vi "Tubing_Corrections_17.vi"() -> (5 "Plug in titles":string[](array[string]), 7 "Plug in values":string[](array[string]))   [LabVIEW 2010]
uses:
  Globals/Meas_global.vi
  <vilib>/Analysis/NI_AALPro.lvlib
  <vilib>/Utility/file.llb/Read From Spreadsheet File (DBL).vi
  <vilib>/Analysis/2dsp.llb/Inverse Real FFT.vi
panel:
  in  "Use a Smoothed\nAverage ITF?":u16(ring) caption="Save Data?" items=["Yes", "No"]
  out "Analogue Out":dbl[][](array[numeric])
  in  "Analogue In":dbl[][](array[numeric])
  in  "Top Level Folder":path
  in  "Use a DC Mag. of 1?":u16(ring)=1 caption="Save Data?" items=["Yes", "No"]
  out "Maximum frequency used from ITF <= Frequency covered in ITF":bool
  in  "Max.  Freq. covered in ITF":dbl=10000.0
  out "No. of samples used is an even no.":bool
  in  "Transducer\nZero Reading":dbl format="%#_p"
  in  "Inv Trans Function":u16(ring) caption="Save Data?" items=["Lee", "RWDI"]
  out "Pressure Signal":cluster{"Y":dbl[], "Y":dbl[]}[](graph)
  out "No. of samples used is constant throughout":bool
  out "Frequency of data used = as taken from the ITF":bool
  out "No. of samples per block\ntaken from raw data":dbl
  in  "Max.  Freq. required from ITF":dbl=10000.0
  in  "Distorted Pressure Channel:":dbl=2.0
  out "No. of samples recorded in raw data = as requested":bool
  in  "Tube Length":u16(ring)=1800 items=["0 mm"=0, "1100 mm"=1100, "1200 mm"=1200, "1300 mm"=1300, "1400 mm"=1400, "1500 mm"=1500, "1600 mm"=1600, "1700 mm"=1700, "1800 mm"=1800, "1900 mm"=1900, "2000 mm"=2000, "2100 mm"=2100, "2200 mm"=2200, "2300 mm"=2300, "2400 mm"=2400, "2500 mm"=2500, "2600 mm"=2600, "2700 mm"=2700, "2800 mm"=2800]
  out "Processing last block?":bool
  # "PLUG IN VI TO APPLY THE INVERSE TRANSFER FUNCTION TO THE PRESSURE DATA COLLECTED."
  # "NOTE: The run/test that is used in the ITF is read from a spreadsheet file.  Therefore when the best ones are found they can be kept and easily accessed.  If the boxes here are left as zero then they will be ignored even if changing the ITF used."
  # "USER INPUTS:"
  # "NOTE: If an average ITF is being used then input the final block number included in the average in this space here.  If a smoothed average is being used then pit \"YES\" in both the average and smoothed inputs."
  # "NOTE: The first thing in the list in the measurement program is channel 0 and second is 1 etc..., regardless of the channel number on the ADC."
  # "NOTE: The frequency of the raw data collected needs to be a product of the maximum frequency used from the ITF file when a lower ITF frequency is used (probably 1000 Hz like in RWDI's) than that of the sampling frequency of the collected pressure.  This is so this 'plug-in' can easily take the number of samples required.  If all of the samples are required then input the sampling frequency as the frequency required from the ITF!"
  # "NOTE: The raw data to be corrected needs to be sent through an analogue low pass filter before being sent to the ADC.  This must be equal to or lower than the Nyquist frequency (half of the sampling frequency).  This will then determine the max. frequency that can be presented in the form of the spectrum."
  # "NUMBER OF VALUES USED IN SMOOTHING THE AVERAGE SPECTRA (FiOR THIS GRAPH ONLY!!)"
  # "NOTE: If you don't put all of the blocks in the same file then it won't try to append to old files"
  # "NOTE: If the transfer function is to be changed and the effect on the RMS and spectra is to be analysed then the user can append as many runs as they like to the RMS and Spectra files by altering the relevant input here."
  # "SAVE BLOCKS BETWEEN:"
  # "AND"
  # "OUTPUTS:"
  # "NOTE: If you only want one block, just put the block number in both of the boxes shown here"
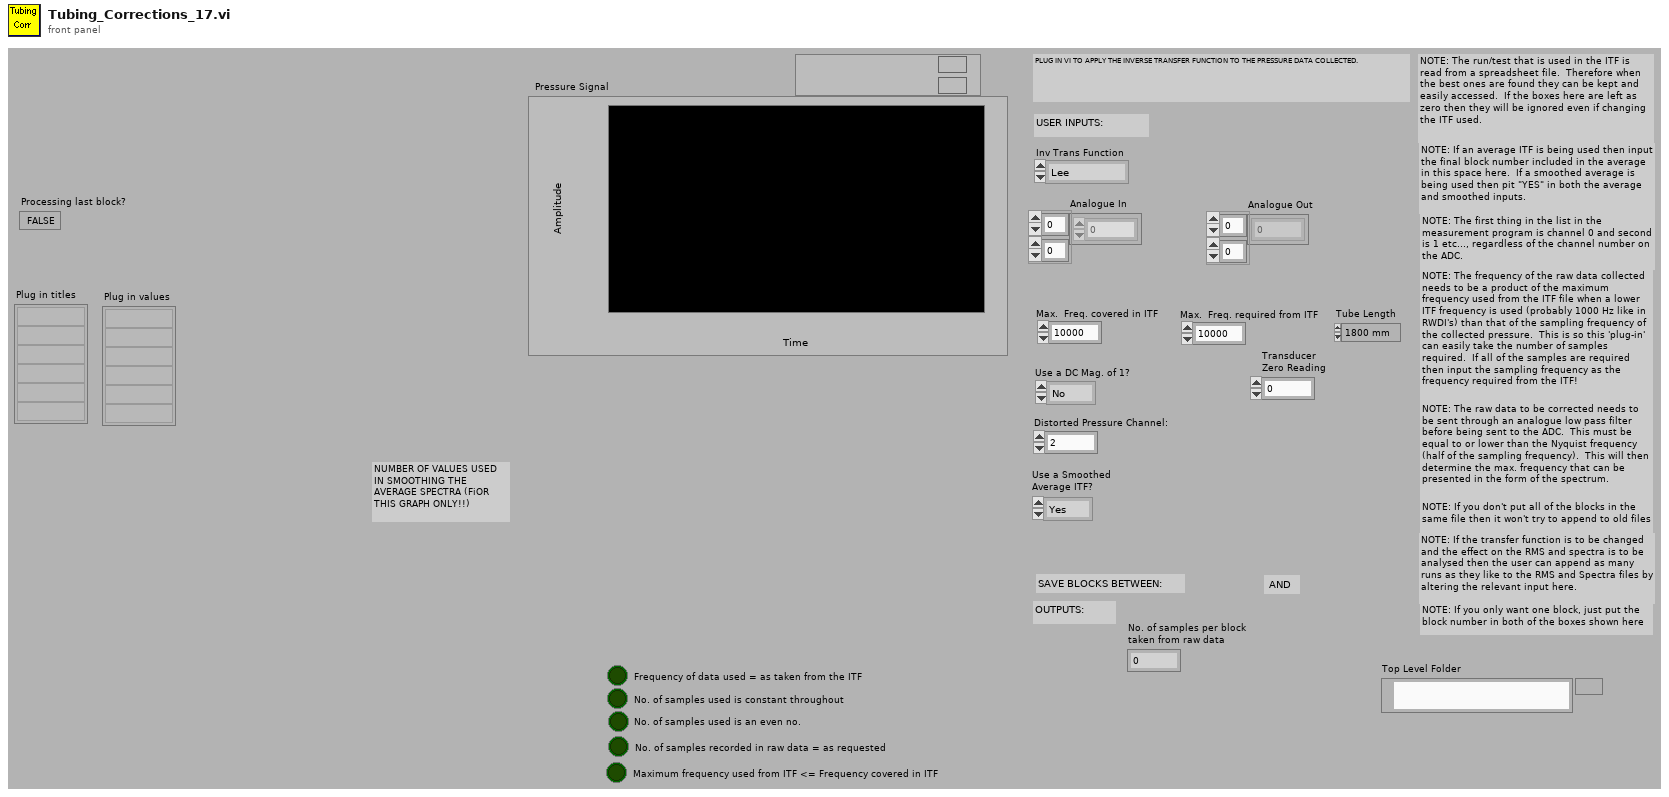
[diagram p1: front panel]
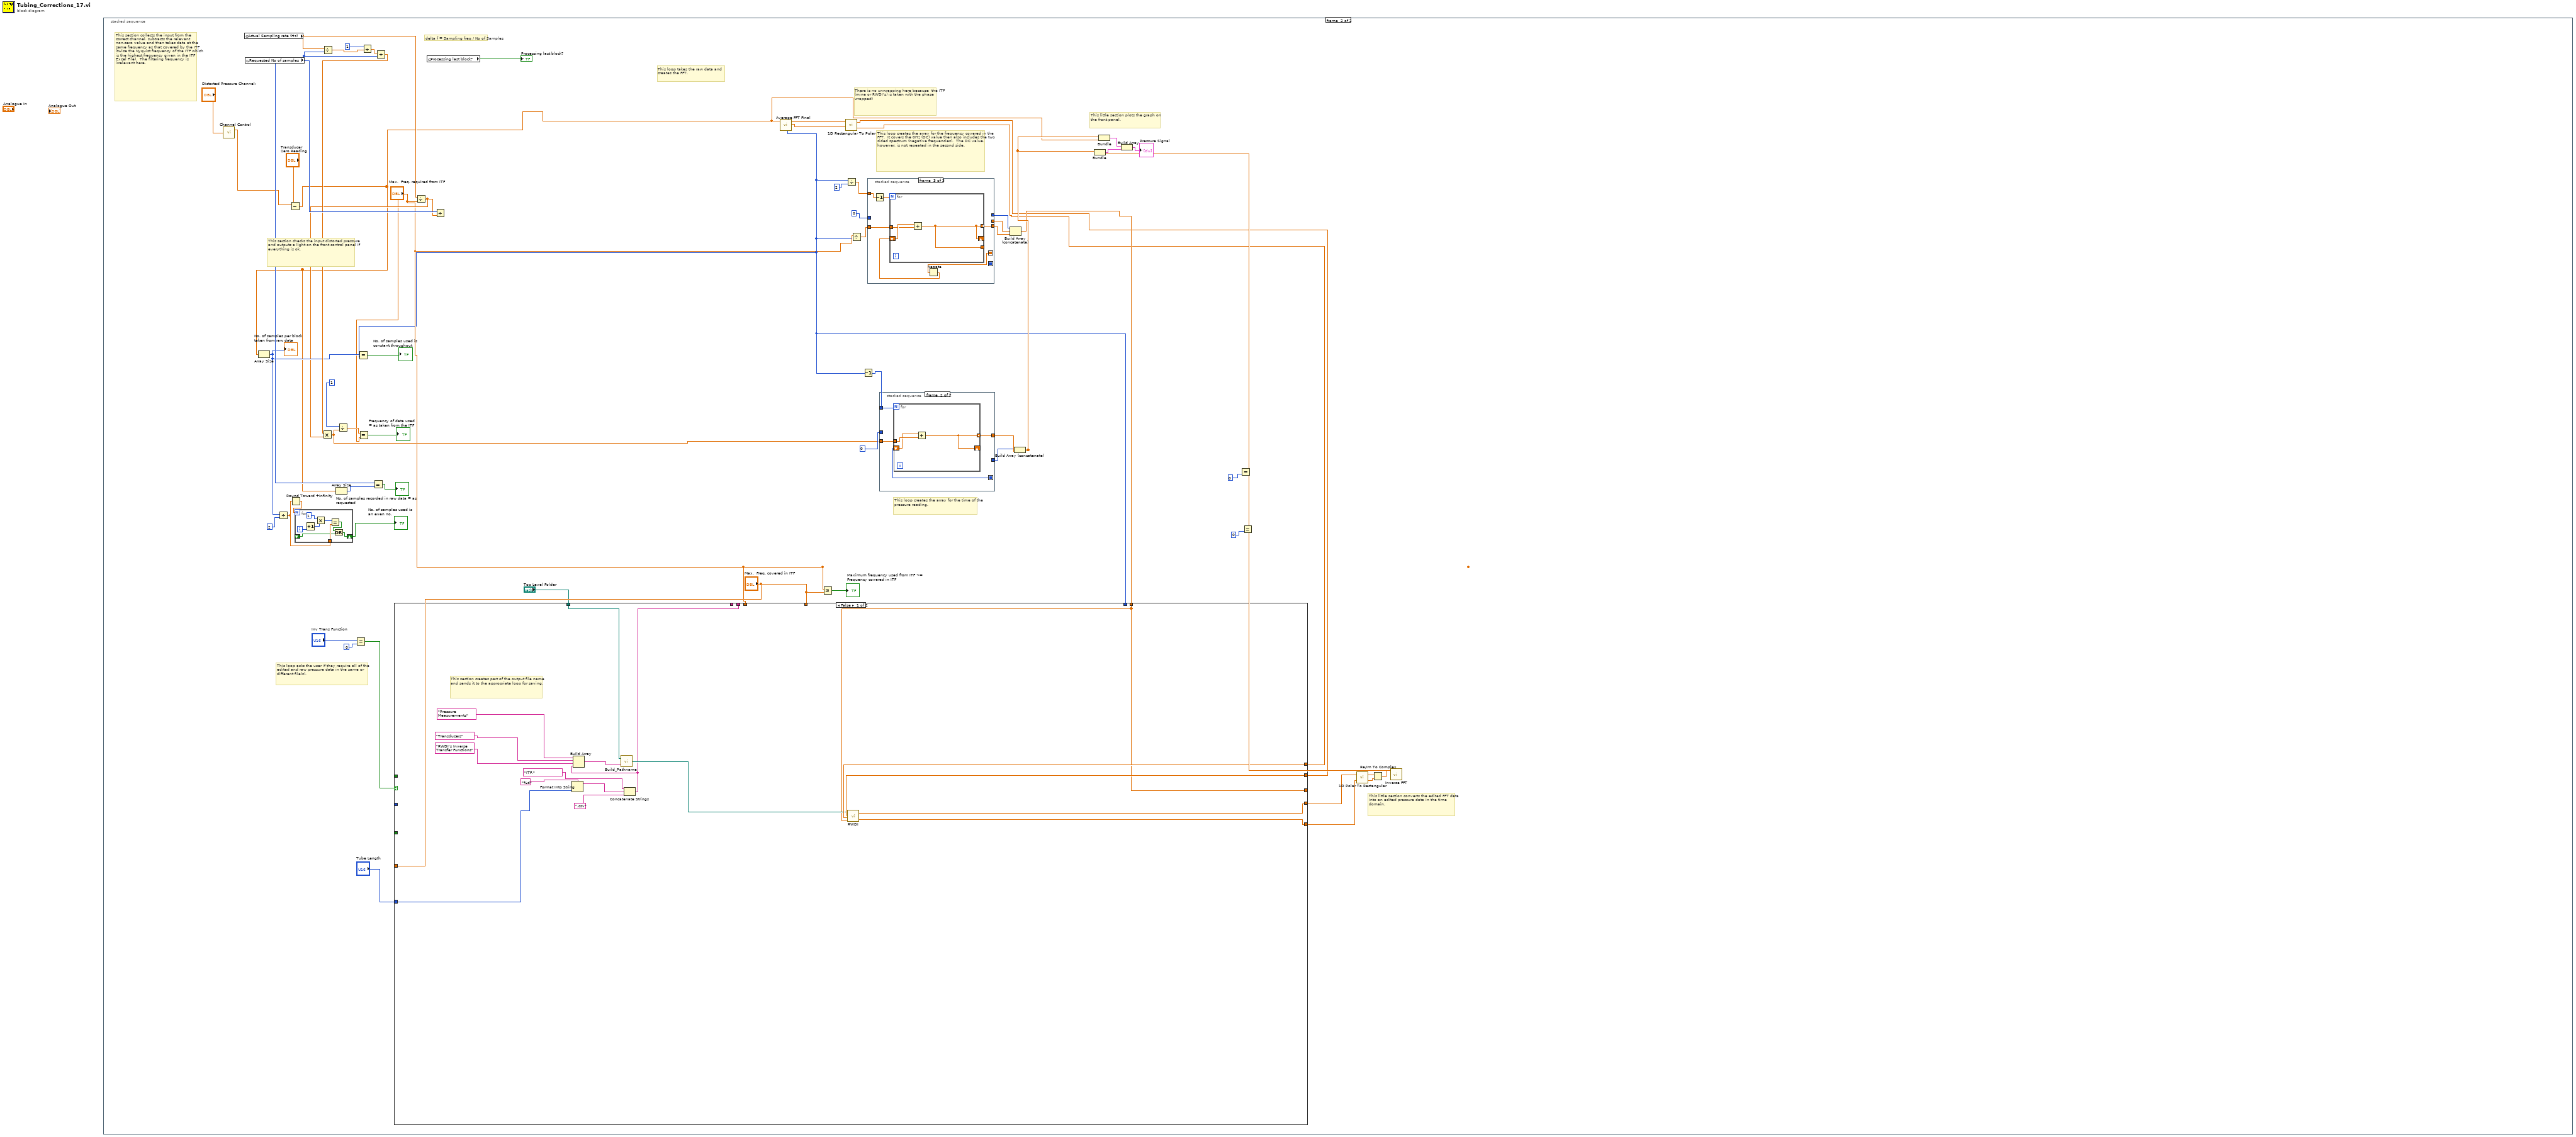
[diagram p0: block diagram]
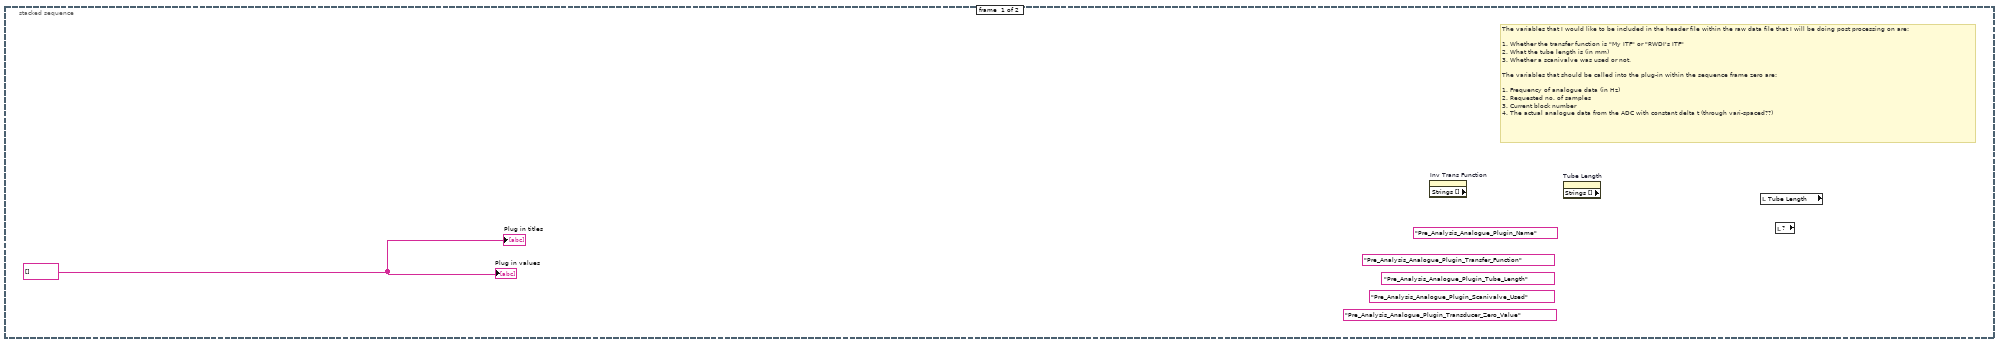
[diagram p2: hidden frame]
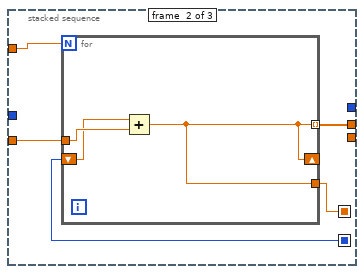
[diagram p4: hidden frame]
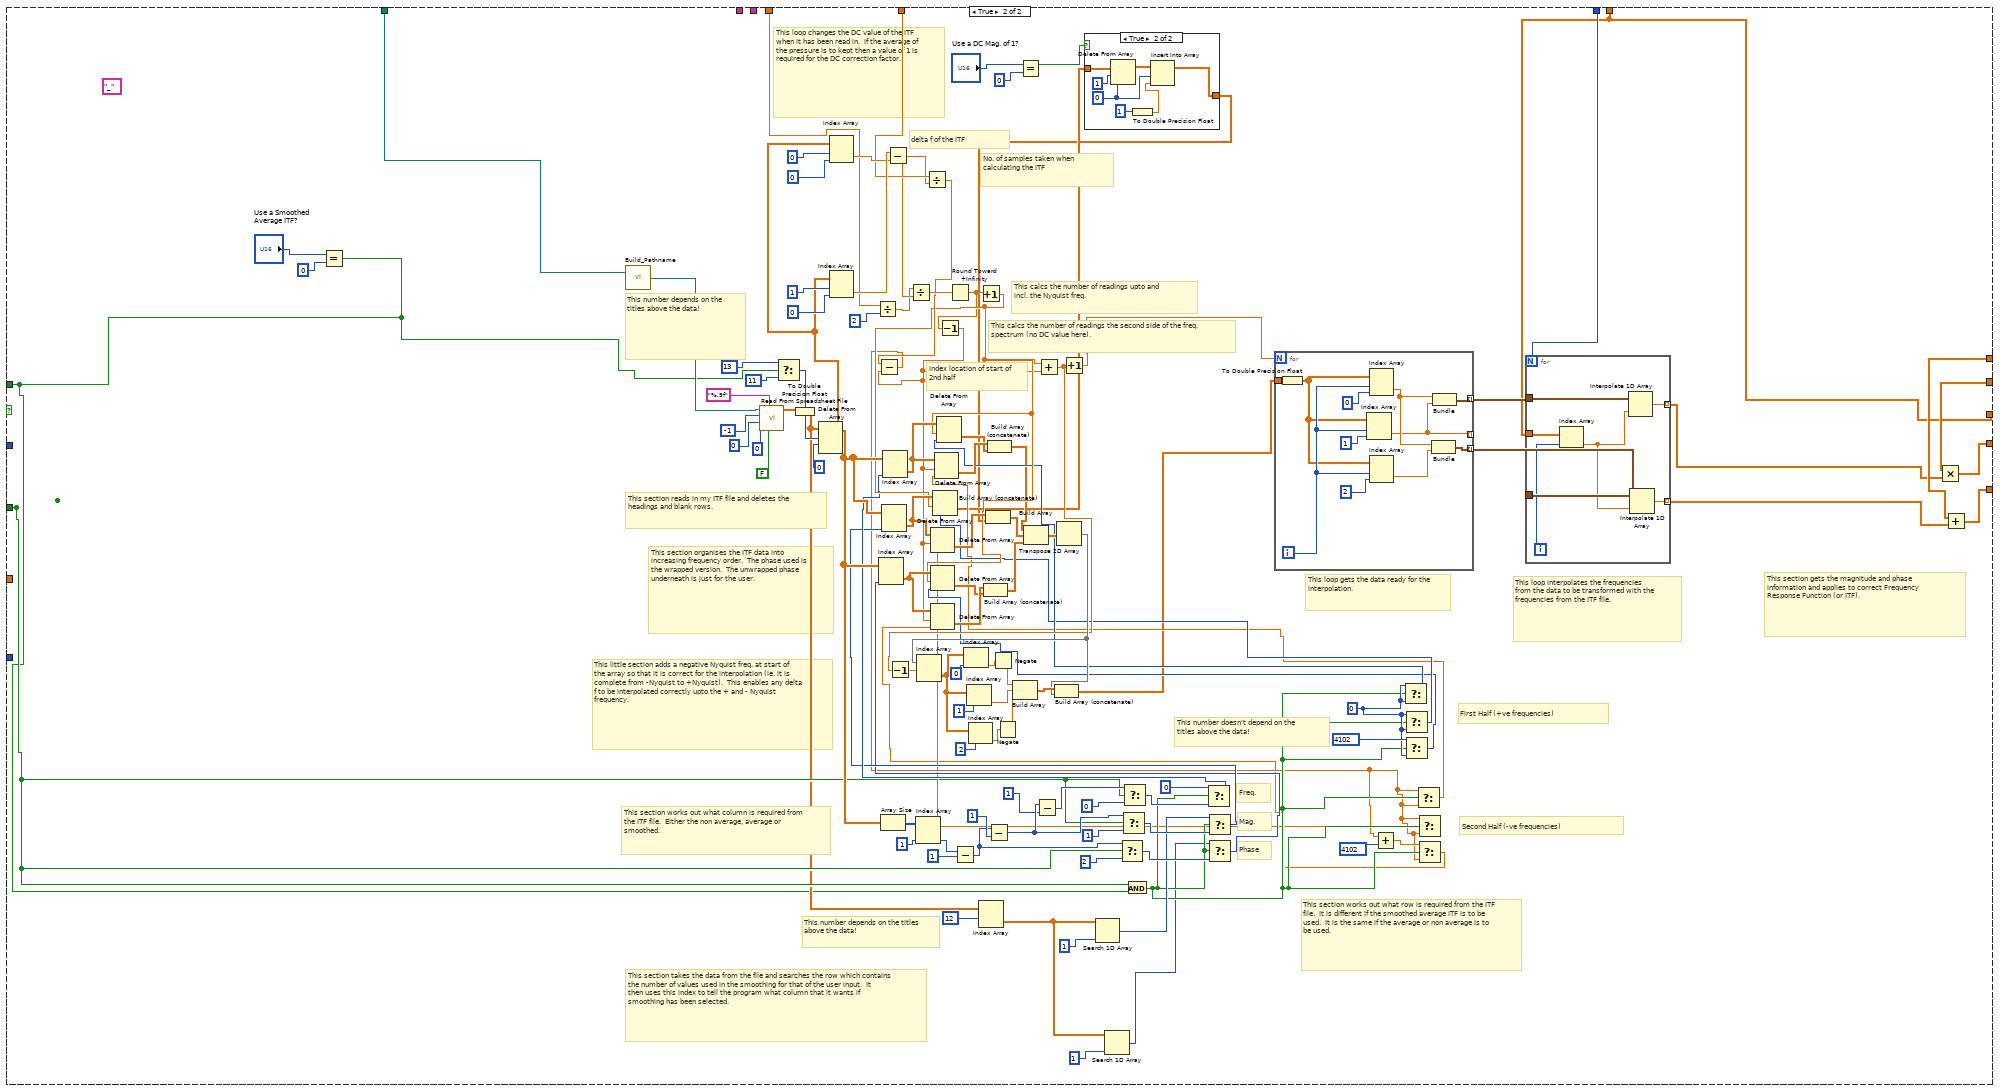
[diagram p5: hidden frame]
diagram:
  n1 = stacked-sequence {
    frame #0 {
      (unwired) "Pre_Analysis_Analogue_Plugin_Transducer_Zero_Value"
      (unwired) "Pre_Analysis_Analogue_Plugin_Scanivalve_Used"
      (unwired) "Pre_Analysis_Analogue_Plugin_Tube_Length"
      (unwired) "Pre_Analysis_Analogue_Plugin_Name"
      (unwired) "Pre_Analysis_Analogue_Plugin_Transfer_Function"
      w1 = string[] [] ("Add in values")
      # "The variables that I would like to be included in the header file within the raw data file that I will be doing post processing on are:\n\n1. Whether the transfer function is \"My ITF\" or \"RWDI's ITF\"\n2. What the tube length is (in mm)\n3. Whether a scanivalve was used or not.\n\nThe variables that should be called into the plug-in within the sequence frame zero are:\n\n1. Frequency of analogue data (in Hz)\n2. Requested no. of samples\n3. Current block number\n4. The actual analogue data from the ADC with constant delta t (through vari-spaced??)"
      n2 = property on="Inv Trans Function" class="Ring (strict)" props=["Strings []"]() -> ()  [unwired: 2 in, 3 out]
      n3 = property on="Tube Length" class="Ring (strict)" props=["Strings []"]() -> ()  [unwired: 2 in, 3 out]
      n4 = local read "Tube Length"() -> ()  [unwired: 1 out]
      n5 = local read item#-1() -> ()  [unwired: 1 out]
      "Plug in titles" <- w1
      "Plug in values" <- w1
    }
    frame #1 {
      # "This little section converts the edited FFT data into an edited pressure data in the time domain."
      # "There is no unwrapping here because  the ITF (mine or RWDI's) is taken with the phase wrapped!"
      # "This loop creates the array for the time of the pressure reading."
      # "This loop creates the array for the frequency covered in the FFT.  It covers the 0Hz (DC) value then also includes the two sided spectrum (negative frequencies).  The DC value, however, is not repeated in the second side."
      # "This loop takes the raw data and creates the FFT."
      # "This section collects the input from the correct channel, subtracts the relevant non-zero value and then takes data at the same frequency as that covered by the ITF (twice the Nyquist frequency of the ITF which is the highest frequency given in the ITF Excel File).  The filtering frequency is irrelevant here."
      # "This section checks the input distorted pressure and outputs a light on the front control panel if everything is ok."
      # "This little section plots the graph on the front panel."
      # "This loop asks the user if they require all of the edited and raw pressure data in the same or different file(s)."
      # "delta f = Sampling freq / No of Samples"
      n6 = call "Channel Control.vi"("Distorted Pressure Channel"="Distorted Pressure Channel:") -> ("Distorted Raw Data"=w10:dbl[])  [unwired: 1 out]
      n7 = global read "Meas_global.vi" "Actual Sampling rate (Hz)"() -> (w60:dbl)
      n8 = global read "Meas_global.vi" "Requested No of samples"() -> (w55:i32)
      n9 = Subtract(x=w10, y="Transducer\nZero Reading") -> (x-y=w5:dbl[])
      n10 = Array Size(array=w5) -> (size(s)=w23:i32)
      "No. of samples per block\ntaken from raw data" <- w23
      n11 = Divide(x=w23, y=2) -> (x/y=w24:dbl)
      n12 = Round Toward +Infinity(x=w24) -> (ceil(x): smallest int >= x=w27:dbl)
      n13 = for {
        N: w27 -> [_]
        tunnel: w24 -> [w75]
        shift-right: [w72] -> w26
        shift-left: _ -> [w73]
        i -> [w79]
        n14 = Increment(x=w79) -> (x+1=w78:i32)
        n15 = Multiply(x=1, y=w78) -> (x*y=w76:i32)
        n16 = Equal?(x=w76, y=w75) -> (x = y?=w74:bool)
        n17 = Or(x=w74, y=w73) -> (x .or. y?=w72:bool)
      }
      "No. of samples used is an even no." <- w26
      n18 = Divide(x=w60, y=w55) -> (x/y=w61:dbl)
      n19 = Array Size(array=w5) -> (size(s)=w54:i32)
      n20 = Equal?(x="Inv Trans Function", y=0) -> (x = y?=w36:bool)
      n21 = Divide(x=1, y=w61) -> (x/y=w59:dbl)
      n22 = Equal?(x=w55, y=w54) -> (x = y?=→"No. of samples recorded in raw data = as requested":bool)
      n23 = Divide(x=w59, y=w55) -> (x/y=w49:dbl)
      n24 = Divide(x=w60, y="Max.  Freq. required from ITF") -> (x/y=w21:dbl)
      n25 = Multiply(x=w49, y=w21) -> (x*y=w35:dbl)
      n26 = Divide(x=1, y=w35) -> (x/y=w57:dbl)
      n27 = Equal?(x=w57, y="Max.  Freq. required from ITF") -> (x = y?=→"Frequency of data used = as taken from the ITF":bool)
      n28 = global read "Meas_global.vi" "Processing last block?"() -> (→"Processing last block?":bool)
      n29 = Divide(x=w55, y=w21) -> ()  [unwired: 1 out]
      n30 = call "Average FFT Final.vi"("Distorted Pressure"=w5) -> ("Spectrum output Imaginary array"=w7:dbl[], "Spectrum output Real array"=w8:dbl[], "No of samples"=w6:i32)  [unwired: 7 in]
      n31 = Equal?(x=w23, y=w6) -> (x = y?=→"No. of samples used is constant throughout":bool)
      n32 = Less Or Equal?(x="Max.  Freq. required from ITF", y="Max.  Freq. covered in ITF") -> (x <= y?=→"Maximum frequency used from ITF <= Frequency covered in ITF":bool)
      n33 = call <vilib>:"1D Rectangular To Polar.vi"("X"=w8, "Y"=w7) -> ("Magnitude"=w3:dbl[], "Phase"=w2:dbl[])  [unwired: 1 out]
      n34 = Divide(x=w6, y=2) -> (x/y=w31:dbl)
      n35 = Divide(x="Max.  Freq. required from ITF", y=w6) -> (x/y=w33:dbl)
      n36 = Decrement(x=w6) -> (x-1=w66:i32)
      n37 = stacked-sequence {
        seq-local: [w80 _ _] -> [_ w84 _]
        seq-local: [_ w83 _] -> [_ _ w92]
        tunnel: 0 -> [w80 _ _]
        tunnel: w33 -> [_ w85 w94]
        tunnel: w31 -> [_ w82 w90]
        tunnel: [_ w81 _] -> w29
        tunnel: [w80 _ _] -> w30
        tunnel: [_ _ w93] -> w28
        frame #0 {
        }
        frame #1 {
          n38 = for {
            N: w82 -> [_]
            tunnel: w85 -> [w88]
            tunnel: [w86] -> w81 mode=indexing
            shift-right: [w86] -> _
            shift-left: w84 -> [w87]
            tunnel: [w86] -> w83
            n39 = Add(x=w87, y=w88) -> (x+y=w86:dbl)
          }
        }
        frame #2 {
          n40 = Decrement(x=w90) -> (x-1=w89:dbl)
          n41 = Negate(x=w92) -> (-x=w91:dbl)
          n42 = for {
            N: w89 -> [_]
            tunnel: [w95] -> w93 mode=indexing
            shift-right: [w95] -> _
            shift-left: w91 -> [w97]
            tunnel: [w95] -> _
            tunnel: w94 -> [w96]
            n43 = Add(x=w97, y=w96) -> (x+y=w95:dbl)
          }
        }
      }
      n44 = stacked-sequence {
        seq-local: [w257 _] -> [_ w258]
        tunnel: 0 -> [w257 _]
        tunnel: w35 -> [_ w260]
        tunnel: w66 -> [_ w261]
        tunnel: [_ w259] -> w65
        tunnel: [w257 _] -> w64
        frame #0 {
        }
        frame #1 {
          n45 = for {
            N: w261 -> [_]
            tunnel: w260 -> [w264]
            tunnel: [w263] -> w259 mode=indexing
            shift-right: [w263] -> _
            shift-left: w258 -> [w262]
            n46 = Add(x=w262, y=w264) -> (x+y=w263:dbl)
          }
        }
      }
      n47 = Build Array (concatenate)(w30, w29, w28) -> (w4:dbl[])
      n48 = case shown="False" w36 {
        tunnel: [_ w127] -> w22
        tunnel: w4 -> [w98 w120]
        tunnel: w2 -> [w112 w224]
        tunnel: w3 -> [w111 w223]
        tunnel: [w98 w120] -> _
        tunnel: [w110 w222] -> w39
        tunnel: [w109 w221] -> w38
        tunnel: w6 -> [_ w197]
        tunnel: [_ w128] -> w37
        tunnel: [w101 _] -> w18
        tunnel: [_ _] -> w13
        tunnel: "Tube Length" -> [w107 _]
        tunnel: "Max.  Freq. covered in ITF" -> [_ _]
        tunnel: "Max.  Freq. covered in ITF" -> [_ w190]
        tunnel: "Max.  Freq. required from ITF" -> [_ w188]
        tunnel: [_ w115] -> w14
        tunnel: "Top Level Folder" -> [w99 w121]
        frame False {
          # "This section creates part of the output file name and sends it to the appropriate loop for saving."
          n49 = Format Into String(format string="%d", w107) -> (resulting string=w108:string)  [unwired: 2 in, 1 out]
          n50 = Concatenate Strings("ITF.", w108, ".csv") -> (w101:string)
          n51 = Build Array("Pressure Measurements", "Transducers", "RWDI's Inverse Transfer Functions", w101) -> (w103:string[])
          n52 = call "Build_Pathname.vi"("Output Array"=w103, "Pathname"=w99) -> ("Appended path"=w102:path)
          n53 = call "RWDI.vi"("Freq"=w98, "Phase In"=w112, "Magnitude In"=w111, "Tranfer_Function_File"=w102) -> ("Phase Out"=w109:dbl[], "Magnitude Out"=w110:dbl[])
        }
        frame True {
          (unwired) "_"
          w150 = 0 ("index (row)")
          # "This loop changes the DC value of the ITF when it has been read in.  If the average of the pressure is to kept then a value of 1 is required for the DC correction factor."
          # "This number depends on the titles above the data!"
          # "This number doesn't depend on the titles above the data!"
          # "This number depends on the titles above the data!"
          # "Phase"
          # "Mag."
          # "Freq."
          # "This section takes the data from the file and searches the row which contains the number of values used in the smoothing for that of the user input.  It then uses this index to tell the program what column that it wants if smoothing has been selected."
          # "Second Half (-ve frequencies)"
          # "First Half (+ve frequencies)"
          # "This section works out what row is required from the ITF file.  It is different if the smoothed average ITF is to be used.  It is the same if the average or non average is to be used."
          # "This little section adds a negative Nyquist freq. at start of the array so that it is correct for the interpolation (ie. it is complete from -Nyquist to +Nyquist).  This enables any delta f to be interpolated correctly upto the + and - Nyquist frequency."
          # "index location of start of 2nd half"
          # "This calcs the number of readings the second side of the freq. spectrum (no DC value here)."
          # "This calcs the number of readings upto and incl. the Nyquist freq."
          # "No. of samples taken when calculating the ITF"
          # "delta f of the ITF"
          # "This section reads in my ITF file and deletes the headings and blank rows."
          # "This section gets the magnitude and phase information and applies to correct Frequency Response Function (or ITF)."
          # "This loop interpolates the frequencies from the data to be transformed with the frequencies from the ITF file."
          # "This loop gets the data ready for the interpolation."
          # "This section works out what column is required from the ITF file.  Either the non average, average or smoothed."
          # "This section organises the ITF data into increasing frequency order.  The phase used is the wrapped version.  The unwrapped phase underneath is just for the user."
          n54 = Equal?(x="Use a Smoothed\nAverage ITF?", y=0) -> (x = y?=w115:bool)
          n55 = call "Build_Pathname.vi"("Pathname"=w121) -> ("Appended path"=w122:path)  [unwired: 1 in]
          n56 = call-poly <vilib>:"Read From Spreadsheet File.vi"("transpose (no:F)"=FALSE, "format (%.3f)"="%.9f", "max characters/row  (no limit:0)"=0, "start of read offset (chars.:0)"=0, "number of rows (all:-1)"=-1, "file path (dialog if empty)"=w122) -> ("all rows"=w124:dbl[][])  [unwired: 1 in, 4 out]
          n57 = Select(t=13 ("index (row)"), s=w115, f=11 ("index (row)")) -> (s? t:f=w125:i32)
          n58 = To Double Precision Float(number=w124) -> (double precision float=w123:dbl[][])
          n59 = Delete From Array(array=w123, length=w125, index (row)=0) -> (array with subset deleted=w189:dbl[][])  [unwired: 1 in, 1 out]
          n60 = Index Array(array=w189, index (row)=0, index (col)=0) -> (element=w191:dbl)
          n61 = Index Array(array=w189, index (row)=1, index (col)=0) -> (element=w192:dbl)
          n62 = Divide(x=w188, y=2) -> (x/y=w185:dbl)
          n63 = Array Size(array=w189) -> (size(s)=w217:i32[])
          n64 = Subtract(x=w192, y=w191) -> (x-y=w186:dbl)
          n65 = Divide(x=w185, y=w186) -> (x/y=w187:dbl)
          n66 = Index Array(array=w217, index #2=1) -> (element #2=w210:i32)  [unwired: 1 in, 1 out]
          n67 = Divide(x=w190, y=w186) -> (x/y=w183:dbl)
          n68 = Round Toward +Infinity(x=w187) -> (ceil(x): smallest int >= x=w180:dbl)
          n69 = Decrement(x=w180) -> (x-1=w181:dbl)
          n70 = Subtract(x=w183, y=w181) -> (x-y=w145:dbl)
          n71 = Subtract(x=w210, y=1 ("disabled index (col)")) -> (x-y=w211:i32)
          n72 = Increment(x=w180) -> (x+1=w182:dbl)
          n73 = Index Array(array=w123, index (row)=12 ("disabled index (col)")) -> (element=w140:dbl[])  [unwired: 1 in]
          n74 = Subtract(x=w211, y=1 ("disabled index (col)")) -> (x-y=w212:i32)
          n75 = Equal?(x="Use a DC Mag. of 1?", y=0) -> (x = y?=w133:bool)
          n76 = Subtract(x=w212, y=1 ("disabled index (col)")) -> (x-y=w213:i32)
          n77 = Add(x=w182, y=w181) -> (x+y=w167:dbl)
          n78 = Decrement(x=w167) -> (x-1=w168:dbl)
          n79 = Increment(x=w167) -> (x+1=w130:dbl)
          n80 = Search 1D Array(1D array=w140, start index (0)=1 ("disabled index (col)")) -> (element=w142:dbl, index of element=w156:i32)
          n81 = Search 1D Array(1D array=w140, start index (0)=1 ("disabled index (col)")) -> (element=w138:dbl, index of element=w139:i32)
          n82 = Select(t=w211, s=w128, f=2 ("disabled index (col)")) -> (s? t:f=w161:i32)
          n83 = Select(t=w212, s=w128, f=1 ("disabled index (col)")) -> (s? t:f=w163:i32)
          n84 = Select(t=w213, s=w128, f=0 ("disabled index (col)")) -> (s? t:f=w165:i32)
          n85 = And(x=w128, y=w115) -> (x .and. y?=w149:bool)
          n86 = Select(t=0 ("index (row)"), s=w149, f=w165) -> (s? t:f=w166:i32)
          n87 = Index Array(array=w189, index (col)=w166) -> (element=w207:dbl[])  [unwired: 1 in]
          n88 = Select(t=w156, s=w149, f=w163) -> (s? t:f=w164:i32)
          n89 = Index Array(array=w189, index (col)=w164) -> (element=w206:dbl[])  [unwired: 1 in]
          n90 = Select(t=w139, s=w149, f=w161) -> (s? t:f=w162:i32)
          n91 = Index Array(array=w189, index (col)=w162) -> (element=w205:dbl[])  [unwired: 1 in]
          n92 = Add(x=w145, y=4102 ("index (row)")) -> (x+y=w146:dbl)
          n93 = Select(t=w150, s=w149, f=w150) -> (s? t:f=w154:i32)
          n94 = Delete From Array(array=w207, length=w182, index=w154) -> (deleted portion=w136:dbl[])  [unwired: 1 out]
          n95 = Select(t=w150, s=w149, f=w150) -> (s? t:f=w153:i32)
          n96 = Delete From Array(array=w206, length=w182, index=w153) -> (deleted portion=w132:dbl[])  [unwired: 1 out]
          n97 = case shown="True" w133 {
            tunnel: w132 -> [w231 w238]
            tunnel: [w231 w232] -> w131
            frame False {
            }
            frame True {
              w235 = 0
              n98 = Delete From Array(array=w238, length=1, index=w235) -> (array with subset deleted=w237:dbl[])  [unwired: 1 out]
              n99 = To Double Precision Float(number=1) -> (double precision float=w233:dbl)
              n100 = Insert Into Array(array=w237, index=w235, new element=w233) -> (w232:dbl[])
            }
          }
          n101 = Select(t=4102 ("index (row)"), s=w149, f=w150) -> (s? t:f=w152:i32)
          n102 = Delete From Array(array=w205, length=w182, index=w152) -> (deleted portion=w201:dbl[])  [unwired: 1 out]
          n103 = Select(t=w145, s=w149, f=w145) -> (s? t:f=w148:dbl)
          n104 = Delete From Array(array=w207, length=w181, index=w148) -> (deleted portion=w204:dbl[])  [unwired: 1 out]
          n105 = Build Array (concatenate)(w204, w136) -> (w137:dbl[])
          n106 = Select(t=w145, s=w149, f=w145) -> (s? t:f=w144:dbl)
          n107 = Delete From Array(array=w206, length=w181, index=w144) -> (deleted portion=w203:dbl[])  [unwired: 1 out]
          n108 = Build Array (concatenate)(w203, w131) -> (w129:dbl[])
          n109 = Select(t=w146, s=w149, f=w145) -> (s? t:f=w143:dbl)
          n110 = Delete From Array(array=w205, length=w181, index=w143) -> (deleted portion=w202:dbl[])  [unwired: 1 out]
          n111 = Build Array (concatenate)(w202, w201) -> (w200:dbl[])
          n112 = Build Array(w137, w129, w200) -> (w198:dbl[][])
          n113 = Transpose 2D Array(2D array=w198) -> (transposed array=w169:dbl[][])
          n114 = Index Array(array=w169, index (row)=w168) -> (element=w176:dbl[])  [unwired: 1 in]
          n115 = Index Array(array=w176, index=0) -> (element=w178:dbl)
          n116 = Index Array(array=w176, index=1) -> (element=w173:dbl)
          n117 = Index Array(array=w176, index=2) -> (element=w172:dbl)
          n118 = Negate(x=w178) -> (-x=w177:dbl)
          n119 = Negate(x=w172) -> (-x=w171:dbl)
          n120 = Build Array(w177, w173, w171) -> (w170:dbl[])
          n121 = Build Array (concatenate)(w170, w169) -> (w126:dbl[][])
          n122 = for {
            N: w130 -> [_]
            tunnel: w126 -> [w256]
            tunnel: [w251] -> w208 mode=indexing
            tunnel: [w253] -> w209 mode=indexing
            tunnel: [w249] -> _ mode=indexing
            i -> [w254]
            n123 = To Double Precision Float(number=w256) -> (double precision float=w252:dbl[][])
            n124 = Index Array(array=w252, index (row)=w254, index (col)=1 ("disabled index (col)")) -> (element=w249:dbl)
            n125 = Index Array(array=w252, index (row)=w254, index (col)=0 ("disabled index (col)")) -> (element=w250:dbl)
            n126 = Index Array(array=w252, index (row)=w254, index (col)=2 ("disabled index (col)")) -> (element=w255:dbl)
            n127 = Bundle(w250, w255) -> (w253:cluster{dbl, dbl})  [unwired: 1 in]
            n128 = Bundle(w250, w249) -> (w251:cluster{dbl, dbl})  [unwired: 1 in]
          }
          n129 = for {
            N: w197 -> [_]
            tunnel: w209 -> [w245]
            tunnel: w208 -> [w239]
            tunnel: w120 -> [w244]
            tunnel: [w241] -> w119 mode=indexing
            tunnel: [w240] -> w118 mode=indexing
            i -> [w243]
            n130 = Index Array(array=w244, index=w243) -> (element=w242:dbl)
            n131 = Interpolate 1D Array(1:w242, 2:w239) -> (0:w241:dbl)
            n132 = Interpolate 1D Array(1:w242, 2:w245) -> (0:w240:dbl)
          }
          n133 = Multiply(x=w223, y=w119) -> (x*y=w222:dbl[])
          n134 = Add(x=w224, y=w118) -> (x+y=w221:dbl[])
        }
      }
      n135 = Build Array (concatenate)(w64, w65) -> (w42:dbl[])
      n136 = Bundle(w42, w5) -> (w45:cluster{dbl[], dbl[]})  [unwired: 1 in]
      n137 = Equal?(y=0) -> (x=w52:i32, x = y?=w50:bool)
      n138 = Equal?(y=0) -> (x=w47:i32, x = y?=w46:bool)
      n139 = call <vilib>:"1D Polar To Rectangular.vi"("Magnitude"=w39, "Phase"=w38) -> ("X"=w70:dbl[], "Y"=w62:dbl[])  [unwired: 1 out]
      n140 = Re/Im To Complex(1:w62, 2:w70) -> (0:w68:cdb[])
      n141 = call-poly <vilib>:"Inverse FFT.vi"("FFT {X}"=w68) -> ("X"=w12:dbl[])  [unwired: 9 in, 1 out]
      n142 = Bundle(w42, "X"=w12) -> (w44:cluster{dbl[], "X":dbl[]})  [unwired: 1 in]
      n143 = Build Array(w45, w44) -> (→"Pressure Signal":cluster{dbl[], "X":dbl[]}[])
    }
  }
